vi "Test Pipelining.vi"() -> ()   [LabVIEW 2014]
uses:
  <vilib>/Platform/TimedLoop/XDataNode/timing_clust.ctl
  <vilib>/Platform/TimedLoop/XDataNode/nitl_modes.ctl
  <vilib>/Platform/TimedLoop/XDataNode/wakeup.ctl
  <vilib>/rvi/Emulation/niFpgaGetClockAttributes.vi
  <vilib>/rvi/Emulation/niFpgaSctlEmulationGetInTimedLoop.vi
  <vilib>/rvi/Emulation/niFpgaEmulationReportErrorSimple.vi
  <vilib>/rvi/Emulation/niFpgaCriticalErrorInLSC.vi
  <vilib>/Platform/TimedLoop/XDataNode/XDataNode.xnode
  <vilib>/rvi/FXPMathLib/FxpAdd/XNode/nifxpmath_Add.xnode
  <vilib>/rvi/FXPMathLib/FxpMul/XNode/nifxpmath_Multiplier.xnode
  <vilib>/rvi/FXPMathLib/sim/FxpSim.dll
  <vilib>/Platform/TimedLoop/XDataNode/XDNodeRunTimeDep.lvlib
panel:
  out "x+y":fxp<+/-,33,33>
  out "x+y 5":fxp<+,32,32>
  out "x*y":fxp<+,32,32>
  out "x+y 4":fxp<+,32,32>
  out "x+y 3":fxp<+,32,32>
  out "x+y 2":fxp<+,32,32>
  out "i_out":i32
  out "output valid":bool
  out "i":i32
  in  "ArrayIn":i16[](array[numeric])=[0, 0, 0, 0, 0]
  in  "New":bool
  in  "Stop Button":bool
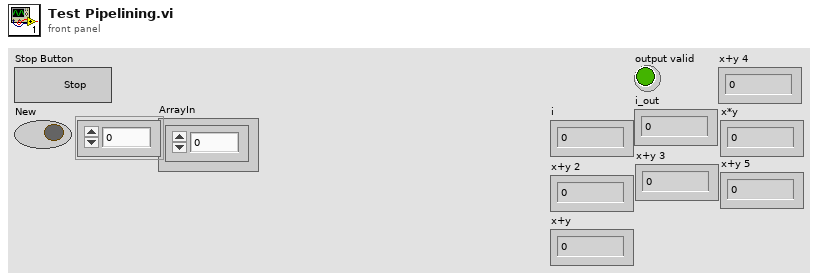
[diagram p1: front panel]
types:
  T1 = typedef "XDNodeRunTimeDep.lvlib/timing_clust.ctl" = cluster{"Expected End [f-1]":u64, "Actual End [f-1]":u64, "Finished Late? [f-1]":bool, "Expected End [i-1]":u64, "Actual End [i-1]":u64, "Finished Late? [i-1]":bool, "Expected Start [i]":u64, "Actual Start [i]":u64, "Expected Start [f]":u64, "Actual Start [f]":u64, "Source Name":string, "Structure Name":string, "Period":i64, "Deadline":i64, "Offset":i64, "Start":i64, "Priority":i32, "Timeout":i32, "Mode":T2, "Wakeup Reason":T3, "Error":errorcluster, "Source Type":string, "Secondary Source Type":string, "Global End Time":u64, "Global Start Time":u64, "Frame Duration":u64, "Iteration Duration":u64, "Assigned CPU":i32, "I/O Scan Engine Mode":u32}
  T2 = typedef "XDNodeRunTimeDep.lvlib/nitl_modes.ctl" = enum32{"No Change", "Process missed periods, maintain original phase", "Discard missed periods, maintain original phase", "Process missed periods, ignore original phase", "Discard missed periods, ignore original phase"}
  T3 = typedef "XDNodeRunTimeDep.lvlib/wakeup.ctl" = enum32{"Normal", "Aborted", "Asynchronous wakeup", "Timing source error", "Timed loop error", "Timeout"}
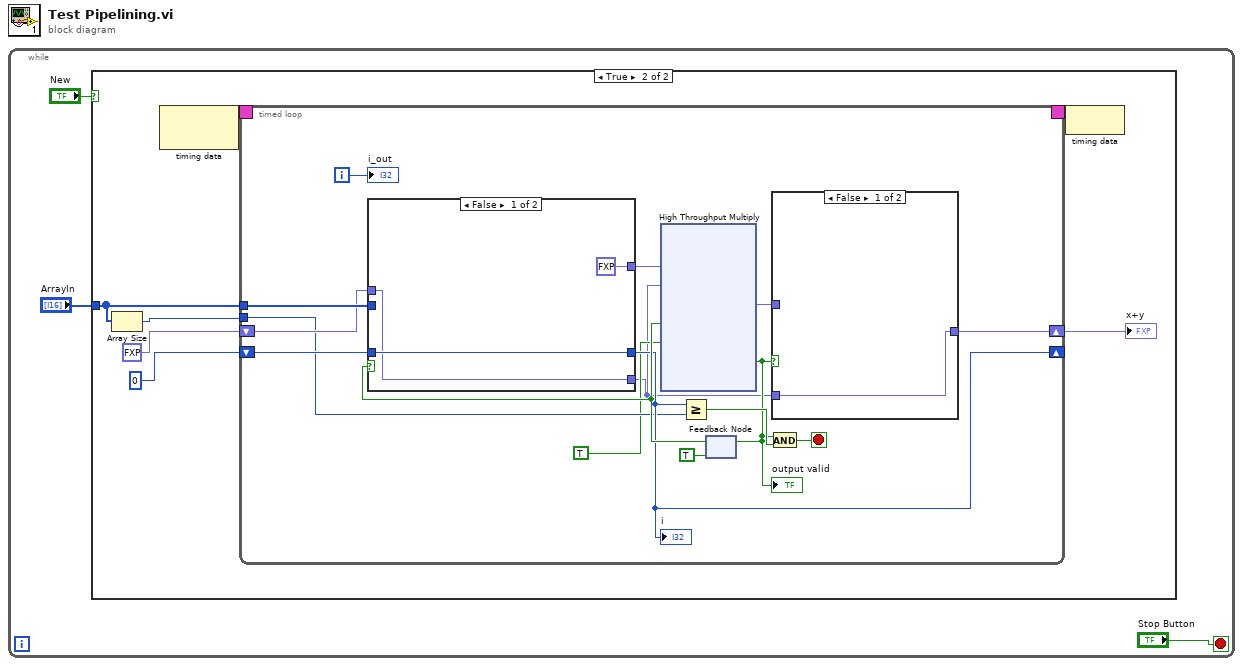
[diagram p0: block diagram]
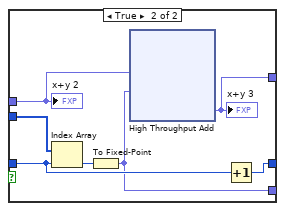
[diagram p3: hidden frame]
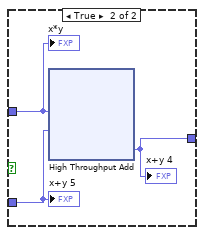
[diagram p4: hidden frame]
diagram:
  n1 = while {
    stop <- "Stop Button" stop-if-true
    n2 = case shown="True" "New" {
      tunnel: "ArrayIn" -> [_ w7]
      frame False {
      }
      frame True {
        n3 = Array Size(array=w7) -> (size(s)=w6:i32)
        n4 = node-c288() -> (w10:T1)  [unwired: 1 in]
        n5 = timed-loop {
          timing: w10 -> [_]
          timing-out: [_] -> w9
          shift-right: [w24] -> w4
          shift-left: fxp<+,32,32> 0.0 ("x+y") -> [w22]
          tunnel: w7 -> [w23]
          shift-right: [w19] -> _
          shift-left: 0 -> [w20]
          tunnel: w6 -> [w18]
          i -> [w14]
          stop <- w15 stop-if-true
          n6 = feedback #1(TRUE ("output valid")) -> (w25:bool)
          n7 = case shown="False" w25 {
            tunnel: [fxp<+,32,32> 0.0 ("x+y") w36] -> w26
            tunnel: w22 -> [w27 w35]
            tunnel: w23 -> [_ w34]
            tunnel: w20 -> [w29 w32]
            tunnel: [w29 w31] -> w19
            tunnel: [w27 w30] -> w11
            frame False {
            }
            frame True {
              n8 = Index Array(array=w34, index=w32) -> (element=w33:i16)
              n9 = To Fixed-Point(number=w33) -> (fixed-point=w30:fxp<+/-,16,16>)  [unwired: 1 in]
              n10 = xnode ("High Throughput Add")("x"=w35, "y"=w30) -> ("x+y"=w36:fxp<+,32,32>)
              "x+y 3" <- w36
              n11 = Increment(x=w32) -> (x+1=w31:i32)
              "x+y 2" <- w35
            }
          }
          "i" <- w19
          n12 = xnode ("High Throughput Multiply")("x"=w26, "y"=w11, "input valid"=w25, "ready for output (T)"=TRUE) -> ("x*y"=w21:fxp<+,32,32>, "output valid"=w16:bool)  [unwired: 1 out]
          "output valid" <- w16
          n13 = Greater Or Equal?(x=w19, y=w18) -> (x >= y?=w17:bool)
          n14 = feedback-in #1(w16) -> ()
          n15 = And(x=w16, y=w17) -> (x .and. y?=w15:bool)
          n16 = case shown="False" w16 {
            tunnel: [w37 w40] -> w24
            tunnel: w11 -> [w37 w38]
            tunnel: w21 -> [_ w39]
            frame False {
            }
            frame True {
              n17 = xnode ("High Throughput Add")("x"=w39, "y"=w38) -> ("x+y"=w40:fxp<+,32,32>)
              "x+y 4" <- w40
              "x*y" <- w39
              "x+y 5" <- w38
            }
          }
          "i_out" <- w14
        }
        "x+y" <- w4
        n18 = node-c288(w9) -> ()
      }
    }
  }
